vi "Messplattenanzeige.vi"(10 "Array":dbl[](array[numeric])) -> ()   [LabVIEW 2015]
panel:
  out "Array 2":dbl[](array[numeric])
  # "Anleitung:\n0-10 ist Platte 1 oder so"
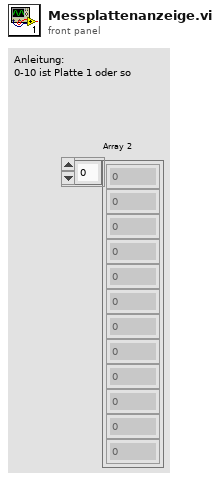
[diagram p1: front panel]
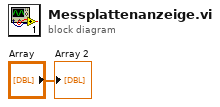
[diagram p0: block diagram]
diagram:
  "Array 2" <- "Array"
